vi "Return_Code_Insertion.vi"(8 "error in (no error)":errorcluster, 11 "Return Code":i32) -> (0 "error out":errorcluster)   [LabVIEW 2013]
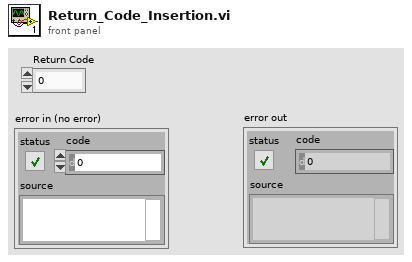
[diagram p1: front panel]
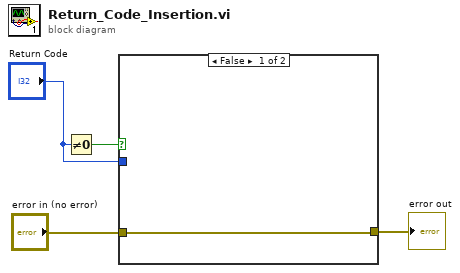
[diagram p0: block diagram]
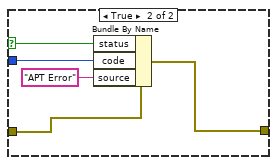
[diagram p2: hidden frame]
diagram:
  n1 = Not Equal To 0?(x="Return Code") -> (x != 0?=w2:bool)
  n2 = case shown="False" w2 {
    selector: w2 -> [_ w8]
    tunnel: "Return Code" -> [_ w7]
    tunnel: "error in (no error)" -> [w5 w10]
    tunnel: [w5 w9] -> w1
    frame False {
    }
    frame True {
      n3 = Bundle By Name(cluster=w10, "status"=w8, "code"=w7, "source"="APT Error") -> (w9:errorcluster)
    }
  }
  "error out" <- w1
